vi "WaveformGraph - Colors.vi"(8 "error in":errorcluster, 10 "Ctl Refnum":refnum<vi>, 11 "Material-Scheme in":refnum<class "Material-Scheme.lvclass">) -> (0 "error out":errorcluster)   [LabVIEW 2021, in "TSC Material Theme.lvlib" / "Material-Scheme.lvclass"]
doc: "Set the colors for a waveform graph type.\n\nColor Rules:\n- Frame, Plot BG: surfaceContainerLowest (preserve transparency)\n- Plot Border: surfaceContainerHighest (preserve transparency)\n- X&Y Scale text: onSurface\n- X&Y Scale gridlines: surfaceContainerHigh (preserve transparency)\n- Plots recolored according to surfaceContainerLowest blending and ratio checking\n- Cursors recolored according to surfaceContainerLowest blending and ratio checking\n\n<b>Code Developed By:</b> +\nDaniel Coons +\nTechnology Service Corporation +\nwww.tsc.com/atcs"
uses:
  Material-Scheme.lvclass
  Material-Scheme.lvclass/Material-Scheme.ctl
  Material SubVIs/Color to HSL.vi
  Material SubVIs/Color to Luminance.vi
  Material SubVIs/HSL to Color.vi
  Material SubVIs/tsc--RGB to Color.vi
  <vilib>/Utility/colorconv.llb/Color to RGB.vi
  Material SubVIs/Material SubVIs.lvlib
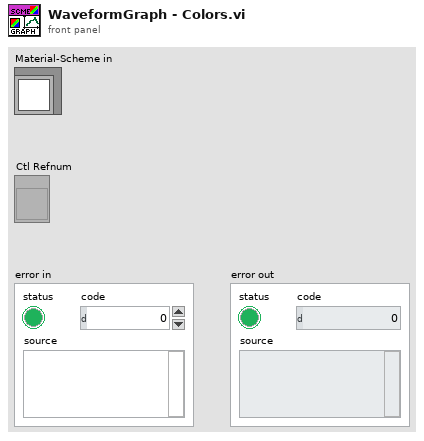
[diagram p1: front panel]
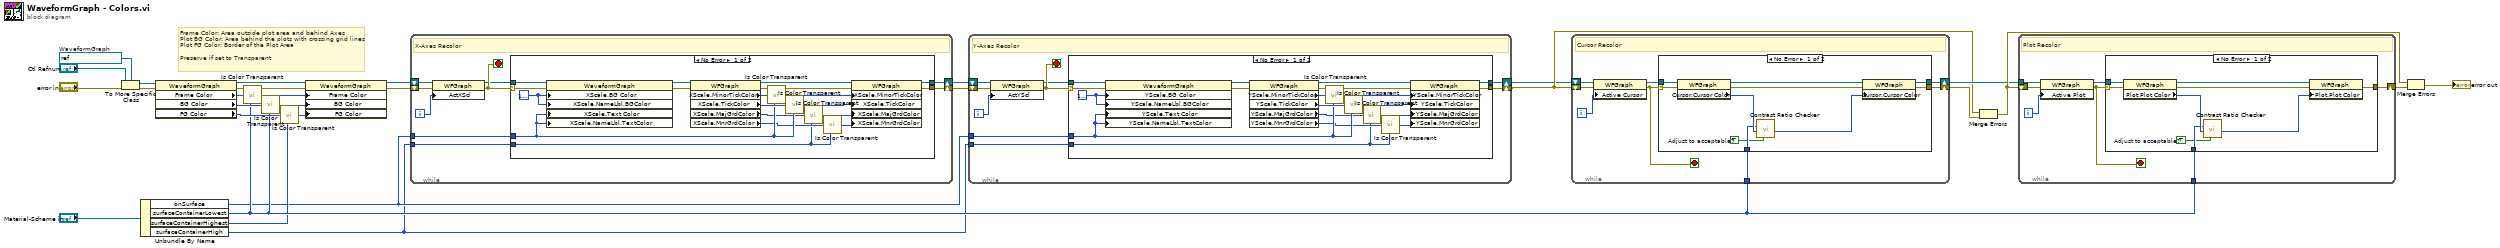
[diagram p0: block diagram]
diagram:
  w24 = refnum<vi> refnum  # WaveformGraph
  # "Frame Color: Area outside plot area and behind Axes\nPlot BG Color: Area behind the plots with crossing grid lines\nPlot FG Color: Border of the Plot Area\n\nPreserve if set to Transparent"
  n1 = To More Specific Class(target class=w24, reference="Ctl Refnum", error in="error in") -> (specific class reference=w8:refnum<vi>, error out=w7:errorcluster)
  n2 = Unbundle By Name("Material-Scheme in") -> ("onSurface"=w4:u32, "surfaceContainerLowest"=w6:u32, "surfaceContainerHighest"=w5:u32, "surfaceContainerHigh"=w3:u32)
  n3 = property class="WaveformGraph"(reference=w8, error in=w7) -> (reference out=w18:refnum<vi>, error out=w19:errorcluster, "Frame Color"=w10:u32, "BG Color"=w11:u32, "FG Color"=w12:u32)
  n4 = call "Is Color Transparent.vi"("original color"=w10, "desired color"=w6) -> ("updated color"=w9:u32)  [unwired: 3 in]
  n5 = call "Is Color Transparent.vi"("original color"=w11, "desired color"=w6) -> ("updated color"=w13:u32)  [unwired: 3 in]
  n6 = call "Is Color Transparent.vi"("original color"=w12, "desired color"=w5) -> ("updated color"=w20:u32)  [unwired: 3 in]
  n7 = property class="WaveformGraph"(reference=w18, error in=w19, "Frame Color"=w9, "BG Color"=w13, "FG Color"=w20) -> (reference out=w16:refnum<vi>, error out=w17:errorcluster)
  n8 = while {
    shift-right: [w34] -> w15
    shift-left: w17 -> [w38]
    tunnel: w4 -> [w32]
    tunnel: w3 -> [w31]
    shift-right: [w30] -> w14
    shift-left: w16 -> [w37]
    i -> [w36]
    stop <- w35 stop-if-true
    # "X-Axes Recolor"
    n9 = property class="WFGraph"(reference=w37, error in=w38, "ActXScl"=w36) -> (reference out=w33:refnum<vi>, error out=w35:errorcluster)
    n10 = case shown="No Error" w35 {
      selector: w35 -> [w57 _]
      tunnel: [w50 _] -> w34
      tunnel: w33 -> [w56 w58]
      tunnel: w32 -> [w46 _]
      tunnel: w31 -> [w40 _]
      tunnel: [w39 w58] -> w30
      frame No Error {
        w55 = u32 16777216 ("X Scale.Name Label.Colors:FG Color")
        n11 = property class="WaveformGraph"(reference=w56, error in=w57, "XScale.BG Color"=w55, "XScale.NameLbl.BGColor"=w55, "XScale.Text Color"=w46, "XScale.NameLbl.TextColor"=w46) -> (reference out=w53:refnum<vi>, error out=w54:errorcluster)
        n12 = property class="WFGraph"(reference=w53, error in=w54) -> (reference out=w51:refnum<vi>, error out=w52:errorcluster, "XScale.MinorTickColor"=w49:u32, "XScale.TickColor"=w47:u32, "XScale.MajGrdColor"=w44:u32, "XScale.MnrGrdColor"=w43:u32)
        n13 = call "Is Color Transparent.vi"("original color"=w49, "desired color"=w46) -> ("updated color"=w48:u32)  [unwired: 3 in]
        n14 = call "Is Color Transparent.vi"("original color"=w47, "desired color"=w46) -> ("updated color"=w45:u32)  [unwired: 3 in]
        n15 = call "Is Color Transparent.vi"("original color"=w44, "desired color"=w40) -> ("updated color"=w42:u32)  [unwired: 3 in]
        n16 = call "Is Color Transparent.vi"("original color"=w43, "desired color"=w40) -> ("updated color"=w41:u32)  [unwired: 3 in]
        n17 = property class="WFGraph"(reference=w51, error in=w52, "XScale.MinorTickColor"=w48, "XScale.TickColor"=w45, "XScale.MajGrdColor"=w42, "XScale.MnrGrdColor"=w41) -> (reference out=w39:refnum<vi>, error out=w50:errorcluster)
      }
      frame Error {
      }
    }
  }
  n18 = while {
    shift-right: [w63] -> w2
    shift-left: w15 -> [w67]
    tunnel: w4 -> [w61]
    tunnel: w3 -> [w60]
    shift-right: [w59] -> w1
    shift-left: w14 -> [w66]
    i -> [w65]
    stop <- w64 stop-if-true
    # "Y-Axes Recolor"
    n19 = property class="WFGraph"(reference=w66, error in=w67, "ActYScl"=w65) -> (reference out=w62:refnum<vi>, error out=w64:errorcluster)
    n20 = case shown="No Error" w64 {
      selector: w64 -> [w86 _]
      tunnel: [w79 _] -> w63
      tunnel: w62 -> [w85 w87]
      tunnel: w61 -> [w75 _]
      tunnel: w60 -> [w69 _]
      tunnel: [w68 w87] -> w59
      frame No Error {
        w84 = u32 16777216 ("X Scale.Name Label.Colors:FG Color")
        n21 = property class="WaveformGraph"(reference=w85, error in=w86, "YScale.BG Color"=w84, "YScale.NameLbl.BGColor"=w84, "YScale.Text Color"=w75, "YScale.NameLbl.TextColor"=w75) -> (reference out=w82:refnum<vi>, error out=w83:errorcluster)
        n22 = property class="WFGraph"(reference=w82, error in=w83) -> (reference out=w80:refnum<vi>, error out=w81:errorcluster, "YScale.MinorTickColor"=w78:u32, "YScale.TickColor"=w76:u32, "YScale.MajGrdColor"=w73:u32, "YScale.MnrGrdColor"=w72:u32)
        n23 = call "Is Color Transparent.vi"("original color"=w78, "desired color"=w75) -> ("updated color"=w77:u32)  [unwired: 3 in]
        n24 = call "Is Color Transparent.vi"("original color"=w76, "desired color"=w75) -> ("updated color"=w74:u32)  [unwired: 3 in]
        n25 = call "Is Color Transparent.vi"("original color"=w73, "desired color"=w69) -> ("updated color"=w71:u32)  [unwired: 3 in]
        n26 = call "Is Color Transparent.vi"("original color"=w72, "desired color"=w69) -> ("updated color"=w70:u32)  [unwired: 3 in]
        n27 = property class="WFGraph"(reference=w80, error in=w81, "YScale.MinorTickColor"=w77, "YScale.TickColor"=w74, "YScale.MajGrdColor"=w71, "YScale.MnrGrdColor"=w70) -> (reference out=w68:refnum<vi>, error out=w79:errorcluster)
      }
      frame Error {
      }
    }
  }
  n28 = while {
    shift-right: [w93] -> w25
    shift-left: w2 -> [w95]
    tunnel: w6 -> [w90]
    shift-right: [w88] -> w21
    shift-left: w1 -> [w89]
    i -> [w92]
    stop <- w94 stop-if-true
    # "Cursor Recolor"
    n29 = property class="WFGraph"(reference=w89, error in=w95, "Active Cursor"=w92) -> (reference out=w91:refnum<vi>, error out=w94:errorcluster)
    n30 = case shown="No Error" w94 {
      selector: w94 -> [w105 _]
      tunnel: [w103 _] -> w93
      tunnel: w91 -> [w102 w106]
      tunnel: w90 -> [w100 _]
      tunnel: [w96 w106] -> w88
      frame No Error {
        w99 = TRUE  # Adjust to acceptable?
        n31 = property class="WFGraph"(reference=w102, error in=w105) -> (reference out=w98:refnum<vi>, error out=w104:errorcluster, "Cursor.Cursor Color"=w101:u32)
        n32 = call "Contrast Ratio Checker.vi"("Adjust to acceptable?"=w99, "On Color"=w101, "Background Color"=w100) -> ("Adjusted Color"=w97:u32)  [unwired: 6 in, 2 out]
        n33 = property class="WFGraph"(reference=w98, error in=w104, "Cursor.Cursor Color"=w97) -> (reference out=w96:refnum<vi>, error out=w103:errorcluster)
      }
      frame Error {
      }
    }
  }
  n34 = Merge Errors(w2, w25) -> (w26:errorcluster)
  n35 = while {
    shift-right: [w111] -> w28
    shift-left: w26 -> [w113]
    tunnel: w6 -> [w108]
    tunnel: w21 -> [w107]
    i -> [w110]
    stop <- w112 stop-if-true
    # "Plot Recolor"
    n36 = property class="WFGraph"(reference=w107, error in=w113, "Active Plot"=w110) -> (reference out=w109:refnum<vi>, error out=w112:errorcluster)
    n37 = case shown="No Error" w112 {
      selector: w112 -> [w122 _]
      tunnel: [w120 _] -> w111
      tunnel: w109 -> [w119 _]
      tunnel: w108 -> [w117 _]
      frame No Error {
        w116 = TRUE  # Adjust to acceptable?
        n38 = property class="WFGraph"(reference=w119, error in=w122) -> (reference out=w115:refnum<vi>, error out=w121:errorcluster, "Plot.Plot Color"=w118:u32)
        n39 = call "Contrast Ratio Checker.vi"("Adjust to acceptable?"=w116, "On Color"=w118, "Background Color"=w117) -> ("Adjusted Color"=w114:u32)  [unwired: 6 in, 2 out]
        n40 = property class="WFGraph"(reference=w115, error in=w121, "Plot.Plot Color"=w114) -> (error out=w120:errorcluster)  [unwired: 1 out]
      }
      frame Error {
      }
    }
  }
  n41 = Merge Errors(w26, w28) -> (→"error out":errorcluster)
